vi "authorRid.get.vi"(8 "error in (no error)":errorcluster, 11 "Run in":refnum<class "Run.lvclass">) -> (0 "error out":errorcluster, 2 "authorRid":string, 3 "Run out":refnum<class "Run.lvclass">)   [LabVIEW 2020, in "Run.lvclass"]
uses:
  Run.lvclass
  Run.lvclass/Run.ctl
  00467254-ce2c-4e37-b69b-d84d91206466.vi
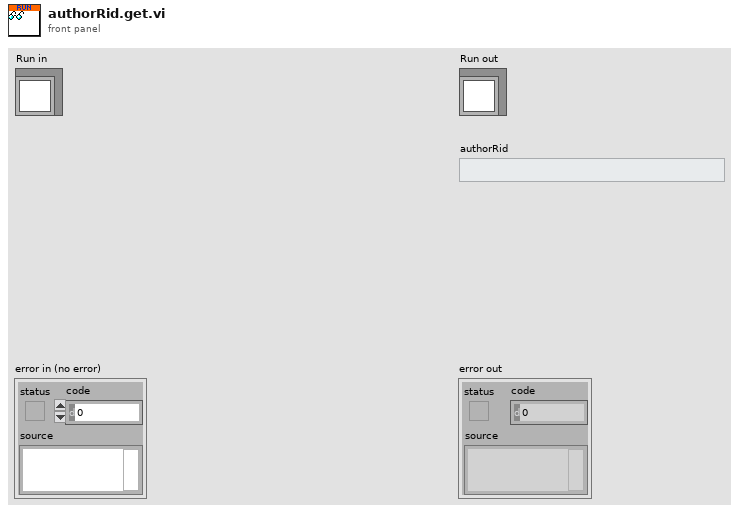
[diagram p1: front panel]
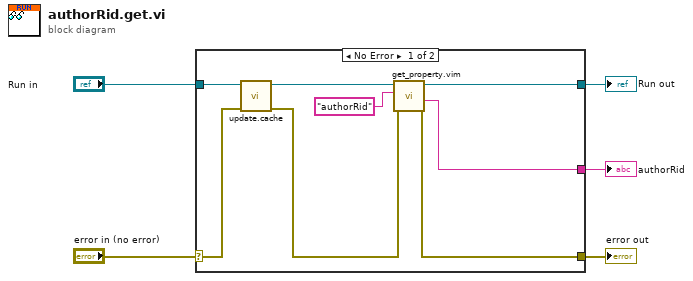
[diagram p0: block diagram]
diagram:
  n1 = case shown="No Error" "error in (no error)" {
    selector: "error in (no error)" -> [w13 w14]
    tunnel: [w6 w14] -> w4
    tunnel: [w8 w15] -> w2
    tunnel: "Run in" -> [w12 w15]
    tunnel: [w10 _] -> w1
    frame No Error {
      n2 = call "update.cache.vi"("error in"=w13, "Run in"=w12) -> ("error out"=w7:errorcluster, "Run out"=w9:refnum<class "Run.lvclass">)  [unwired: 8 in]
      n3 = call "get_property.vim"("error in"=w7, "Property Name"="authorRid", "Run in"=w9) -> ("error out"=w6:errorcluster, "Value"=w10:string, "Run out"=w8:refnum<class "Run.lvclass">)  [unwired: 6 in]
    }
    frame Error {
    }
  }
  "error out" <- w4
  "Run out" <- w2
  "authorRid" <- w1
